vi "Test CPLX EXT Value.vi"(7 "Name":string="Test Complex EXT Value", 9 "Limit":refnum<class "Abs_Complex Extended Float.lvclass">, 10 "Limit Test Type":enum16{"x == Limit", "x != Limit"}(ring), 11 "Tested Value":refnum<class "Abs_Complex Extended Float.lvclass">) -> (3 "abs_Node":refnum<class "abs_Node.lvclass">)   [LabVIEW 2021, in "BT.lvlib"]
uses:
  BT.lvlib
  Support/abs_Node/abs_Node.lvclass
  <vilib>/TSA/Abstract Data Classes/Abs_Types/Complex Extended Float/Abs_Complex Extended Float.lvclass
  C:/Program Files (x86)/National Instruments/LabVIEW 2021/vi.lib/TSA/Abstract Data Classes/Abs_Types/Numeric/Abs_Numeric.lvclass
  Support/Test Boolean/Test Boolean.lvclass
  C:/Program Files (x86)/National Instruments/LabVIEW 2021/vi.lib/TSA/Abstract Data Classes/Abs_Types/Type/Abs_Type.lvclass
  C:/Users/Tim/Documents/GitHub/LV_Behaviour_Tree/Source/Support/abs_Type Leaf/abs_Type Leaf.lvclass
  C:/Users/Tim/Documents/GitHub/LV_Behaviour_Tree/Source/Support/abs_Node/abs_Node.lvclass
  <vilib>/TSA/Abstract Data Classes/Abs_Types/Type/Abs_Type.lvclass/Abs_Type.ctl
  Support/abs_Type Leaf/abs_Type Leaf.lvclass/abs_Type Leaf.ctl
  <vilib>/TSA/Abstract Data Classes/Abs_Types/Type/Properties/Write Name.vi
  Support/abs_Type Leaf/Properties/Write Value Class.vi
  <vilib>/TSA/Abstract Data Classes/Abs_Types/Boolean/Abs_Boolean.lvclass
  <vilib>/TSA/Abstract Data Classes/Functions/Compare/Support/Equal/CPLX_EXT/Method.vi
  <vilib>/TSA/Abstract Data Classes/Functions/Compare/Support/Not Equal/CPLX_EXT/Method.vi
  <vilib>/TSA/Abstract Data Classes/Functions/Compare/Support/Equal/CPLX_EXT/Equal_CPLX_EXT.lvclass
  <vilib>/TSA/Abstract Data Classes/Functions/Compare/Support/Not Equal/CPLX_EXT/Not Equal_CPLX_EXT.lvclass
  C:/Program Files (x86)/National Instruments/LabVIEW 2021/vi.lib/TSA/Abstract Data Classes/Abs_Types/Floating Point/Abs_Floating Point.lvclass
  C:/Program Files (x86)/National Instruments/LabVIEW 2021/vi.lib/TSA/Abstract Data Classes/Abs_Types/Value/Abs_Value.lvclass
  C:/Program Files (x86)/National Instruments/LabVIEW 2021/vi.lib/TSA/Abstract Data Classes/Abs_Types/Complex Extended Float/Abs_Complex Extended Float.lvclass
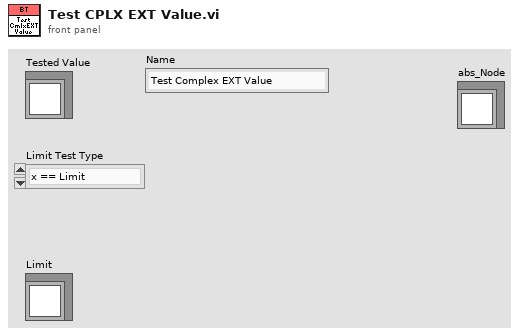
[diagram p1: front panel]
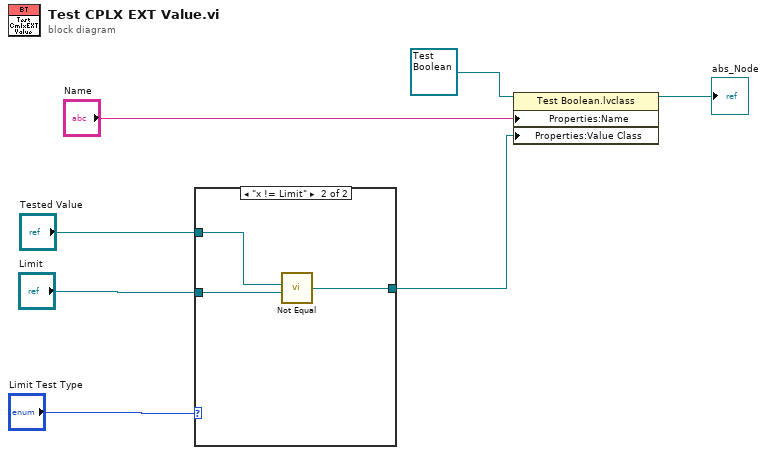
[diagram p0: block diagram]
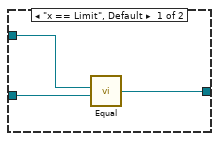
[diagram p2: hidden frame]
diagram:
  n1 = case shown="\"x != Limit\"" "Limit Test Type" {
    tunnel: "Tested Value" -> [w10 w12]
    tunnel: "Limit" -> [w9 w13]
    tunnel: [w8 w11] -> w2
    frame "x == Limit", Default {
      n2 = call-poly <vilib>:"Equal.vi"("Value B"=w9, "Value A"=w10) -> ("Result"=w8:refnum<class "Abs_Boolean.lvclass">)  [unwired: 4 in]
    }
    frame "x != Limit" {
      n3 = call-poly <vilib>:"Not Equal.vi"("Value B"=w13, "Value A"=w12) -> ("Result"=w11:refnum<class "Abs_Boolean.lvclass">)  [unwired: 4 in]
    }
  }
  n4 = property class="Test Boolean.lvclass"(reference=refnum<class "Test Boolean.lvclass"> refnum ("BT.lvlib:Test Boolean.lvclass"), "Properties:Name"="Name", "Properties:Value Class"=w2) -> (reference out=→"abs_Node":refnum<class "Test Boolean.lvclass">)  [unwired: 1 in, 1 out]
